vi "DI IRQ Preview.vi"(6 "Edge Count:":u32, 7 "Type:":T1, 8 "error in (no error)":errorcluster, 9 "_Count Label Refnum":refnum<vi>, 10 "_Counts Refnum":refnum<vi>, 11 "_Digtal Preview Refnum":refnum<vi>) -> (0 "error out":errorcluster)   [LabVIEW 2021]
uses:
  <vilib>/myRIO/Common/Instrument Driver Framework/myRIO v1.0/IRQ/typedefs/DI IRQ Type.ctl
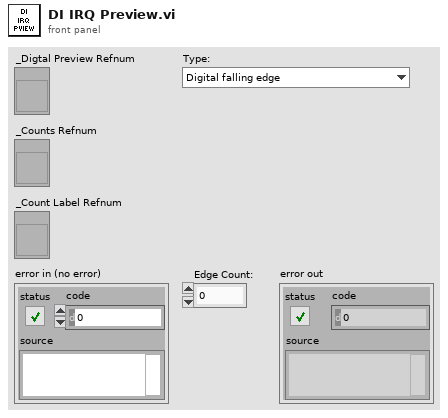
[diagram p1: front panel]
types:
  T1 = typedef "DI IRQ Type.ctl" = enum16{"Digital falling edge", "Digital rising edge", "Digital edge"}
  T2 = cluster{"Analog Preview 3":cluster{"X":dbl, "Y":dbl}[]}[]
  T3 = cluster{"Analog Preview 3":cluster{"X":dbl, "Y":dbl}[]}
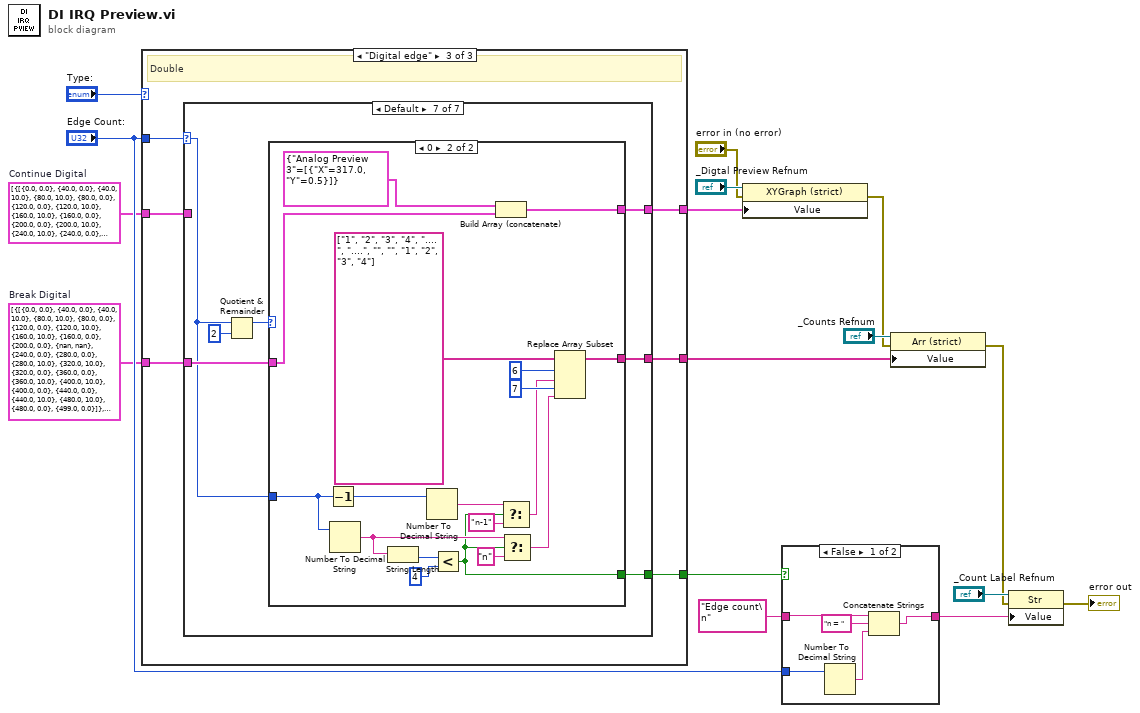
[diagram p0: block diagram]
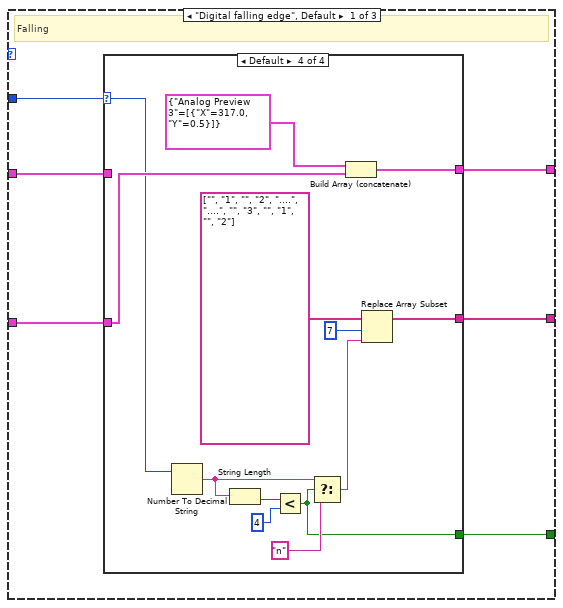
[diagram p3: hidden frame]
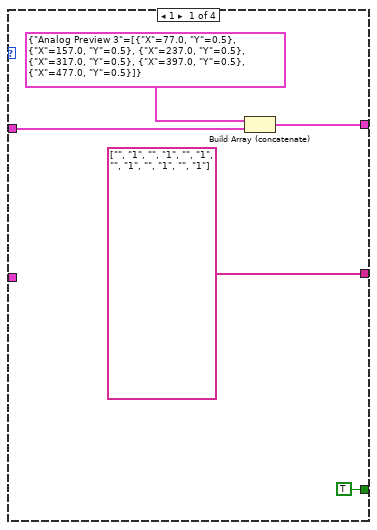
[diagram p4: hidden frame]
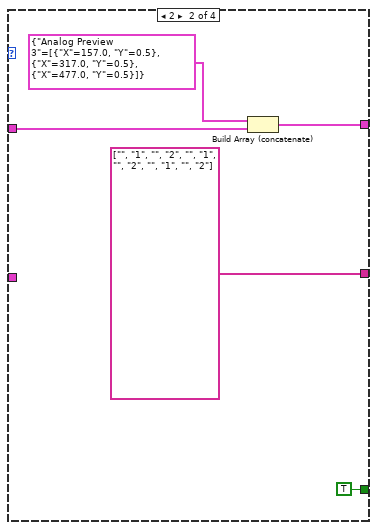
[diagram p5: hidden frame]
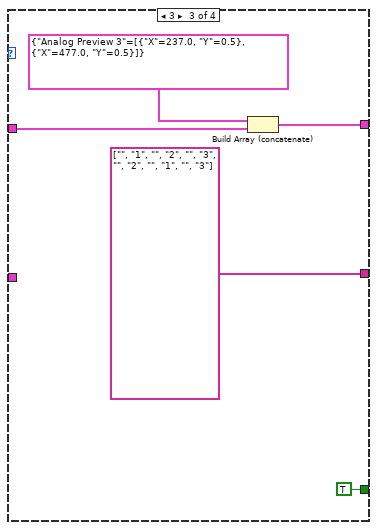
[diagram p6: hidden frame]
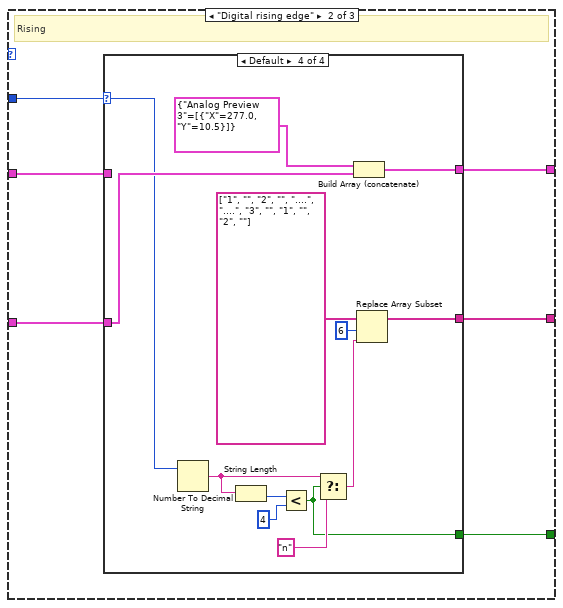
[diagram p7: hidden frame]
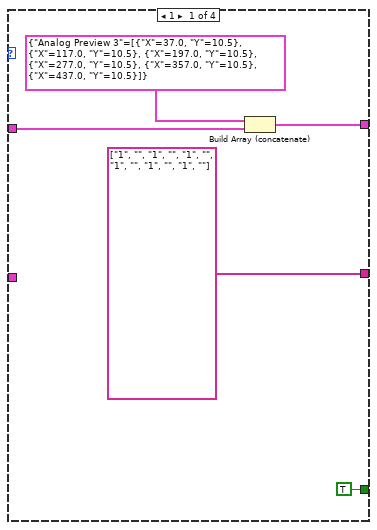
[diagram p8: hidden frame]
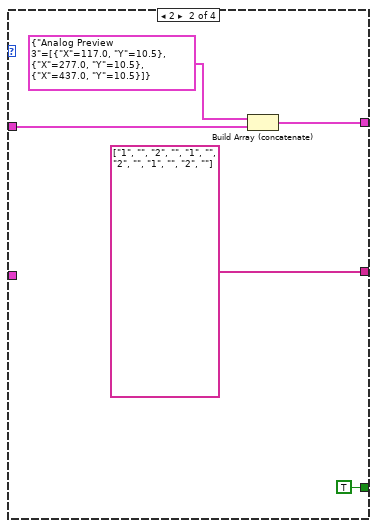
[diagram p9: hidden frame]
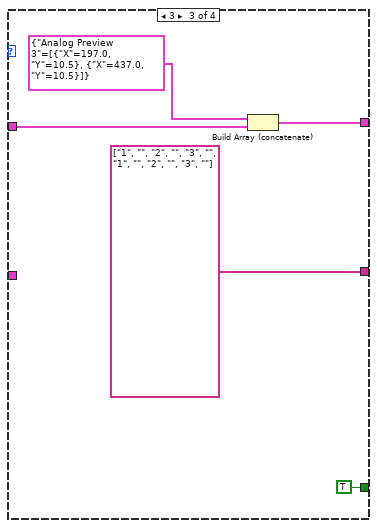
[diagram p10: hidden frame]
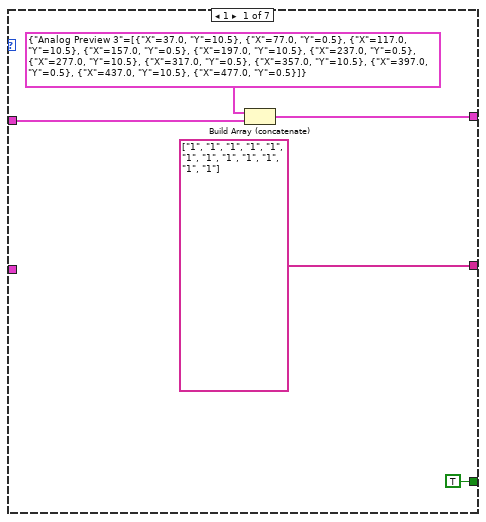
[diagram p11: hidden frame]
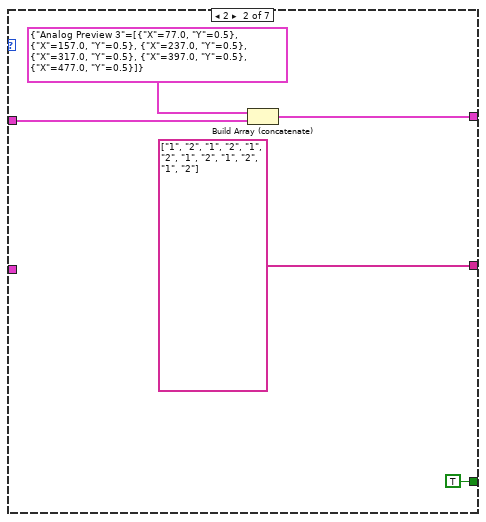
[diagram p12: hidden frame]
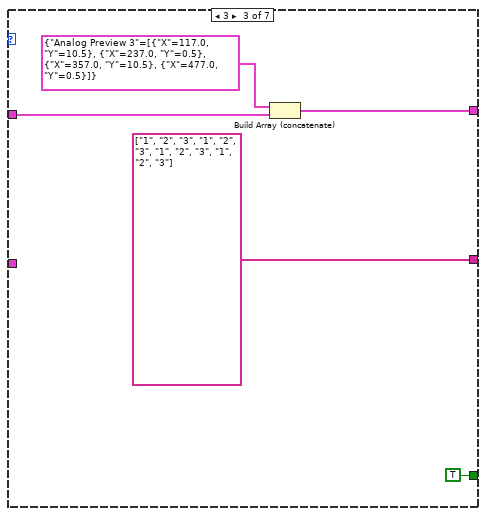
[diagram p13: hidden frame]
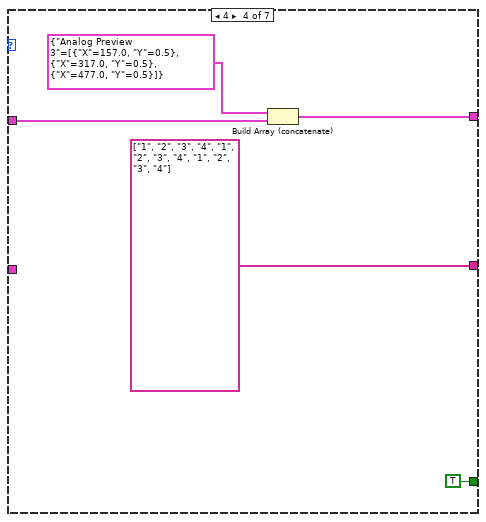
[diagram p14: hidden frame]
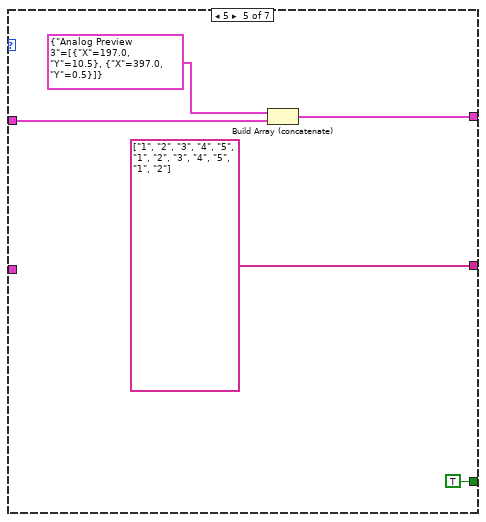
[diagram p15: hidden frame]
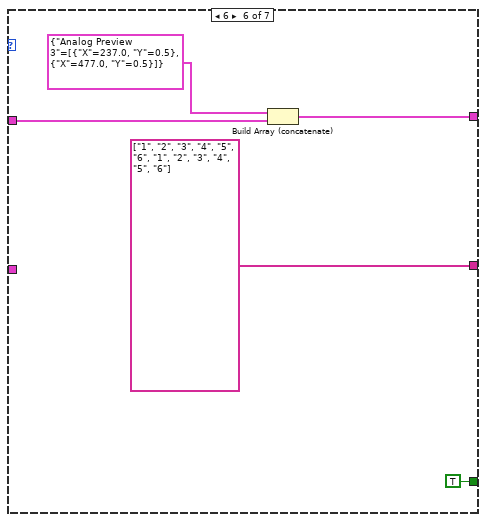
[diagram p16: hidden frame]
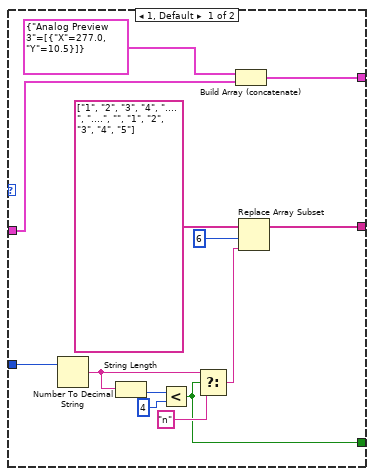
[diagram p17: hidden frame]
diagram:
  w8 = T2 [{"Analog Preview 3"=[{"X"=0.0, "Y"=0.0}, {"X"=40.0, "Y"=0.0}, {"X"=40.0, "Y"=10.0}, {"X"=80.0, "Y"=10.0}, {"X"=80.0, "Y"=0.0}, {"X"=120.0, "Y"=0.0}, {"X"=120.0, "Y"=10.0}, {"X"=160.0, "Y"=10.0}, {"X"=160.0, "Y"=0.0}, {"X"=200.0, "Y"=0.0}, {"X"=nan, "Y"=nan}, {"X"=240.0, "Y"=0.0}, {"X"=280.0, "Y"=0.0}, {"X"=280.0, "Y"=10.0}, {"X"=320.0, "Y"=10.0}, {"X"=320.0, "Y"=0.0}, {"X"=360.0, "Y"=0.0}, {"X"=360.0, "Y"=10.0}, {"X"=400.0, "Y"=10.0}, {"X"=400.0, "Y"=0.0}, {"X"=440.0, "Y"=0.0}, {"X"=440.0, "Y"=10.0}, {"X"=480.0, "Y"=10.0}, {"X"=480.0, "Y"=0.0}, {"X"=499.0, "Y"=0.0}]}, {"Analog Preview 3"=[{"X"=190.0, "Y"=-2.0}, {"X"=200.0, "Y"=0.0}, {"X"=190.0, "Y"=2.0}, {"X"=200.0, "Y"=4.0}, {"X"=nan, "Y"=nan}, {"X"=200.0, "Y"=-2.0}, {"X"=210.0, "Y"=0.0}, {"X"=200.0, "Y"=2.0}, {"X"=210.0, "Y"=4.0}, {"X"=nan, "Y"=nan}, {"X"=220.0, "Y"=-2.0}, {"X"=230.0, "Y"=0.0}, {"X"=220.0, "Y"=2.0}, {"X"=230.0, "Y"=4.0}, {"X"=nan, "Y"=nan}, {"X"=230.0, "Y"=-2.0}, {"X"=240.0, "Y"=0.0}, {"X"=230.0, "Y"=2.0}, {"X"=240.0, "Y"=4.0}]}]  # Break Digital
  w9 = T2 [{"Analog Preview 3"=[{"X"=0.0, "Y"=0.0}, {"X"=40.0, "Y"=0.0}, {"X"=40.0, "Y"=10.0}, {"X"=80.0, "Y"=10.0}, {"X"=80.0, "Y"=0.0}, {"X"=120.0, "Y"=0.0}, {"X"=120.0, "Y"=10.0}, {"X"=160.0, "Y"=10.0}, {"X"=160.0, "Y"=0.0}, {"X"=200.0, "Y"=0.0}, {"X"=200.0, "Y"=10.0}, {"X"=240.0, "Y"=10.0}, {"X"=240.0, "Y"=0.0}, {"X"=280.0, "Y"=0.0}, {"X"=280.0, "Y"=10.0}, {"X"=320.0, "Y"=10.0}, {"X"=320.0, "Y"=0.0}, {"X"=360.0, "Y"=0.0}, {"X"=360.0, "Y"=10.0}, {"X"=400.0, "Y"=10.0}, {"X"=400.0, "Y"=0.0}, {"X"=440.0, "Y"=0.0}, {"X"=440.0, "Y"=10.0}, {"X"=480.0, "Y"=10.0}, {"X"=480.0, "Y"=0.0}, {"X"=499.0, "Y"=0.0}]}]  # Continue Digital
  n1 = case shown="\"Digital edge\"" "Type:" {
    tunnel: "Edge Count:" -> [w22 w56 w86]
    tunnel: w9 -> [w21 w55 w90]
    tunnel: [w19 w54 w88] -> w14
    tunnel: [w18 w53 w87] -> w15
    tunnel: w8 -> [w20 w52 w89]
    tunnel: [w17 w51 w85] -> w11
    frame "Digital falling edge", Default {
      # "Falling"
      n2 = case shown="Default" w22 {
        selector: w22 -> [_ _ _ w40]
        tunnel: w21 -> [w27 w32 w36 _]
        tunnel: [w25 w31 w35 w48] -> w19
        tunnel: [string[] ["", "1", "", "1", "", "1", "", "1", "", "1", "", "1"] ("Count") string[] ["", "1", "", "2", "", "1", "", "2", "", "1", "", "2"] ("Count") string[] ["", "1", "", "2", "", "3", "", "2", "", "1", "", "3"] ("Count") w46] -> w18
        tunnel: w20 -> [_ _ _ w49]
        tunnel: [TRUE TRUE TRUE w38] -> w17
        frame 1 {
          n3 = Build Array (concatenate)(T3 {"Analog Preview 3"=[{"X"=77.0, "Y"=0.5}, {"X"=157.0, "Y"=0.5}, {"X"=237.0, "Y"=0.5}, {"X"=317.0, "Y"=0.5}, {"X"=397.0, "Y"=0.5}, {"X"=477.0, "Y"=0.5}]}, w27) -> (w25:T2)
        }
        frame 2 {
          n4 = Build Array (concatenate)(T3 {"Analog Preview 3"=[{"X"=157.0, "Y"=0.5}, {"X"=317.0, "Y"=0.5}, {"X"=477.0, "Y"=0.5}]}, w32) -> (w31:T2)
        }
        frame 3 {
          n5 = Build Array (concatenate)(T3 {"Analog Preview 3"=[{"X"=237.0, "Y"=0.5}, {"X"=477.0, "Y"=0.5}]}, w36) -> (w35:T2)
        }
        frame Default {
          n6 = Number To Decimal String(number=w40) -> (decimal integer string=w42:string)  [unwired: 1 in]
          n7 = String Length(string=w42) -> (length=w44:i32)
          n8 = Less?(x=w44, y=4) -> (x < y?=w38:bool)
          n9 = Select(t=w42, s=w38, f="n") -> (s? t:f=w39:string)
          n10 = Build Array (concatenate)(T3 {"Analog Preview 3"=[{"X"=317.0, "Y"=0.5}]}, w49) -> (w48:T2)
          n11 = Replace Array Subset(array=string[] ["", "1", "", "2", "....", "....", "", "3", "", "1", "", "2"] ("Count"), new element=w39, index=7) -> (w46:string[])
        }
      }
    }
    frame "Digital rising edge" {
      # "Rising"
      n12 = case shown="Default" w56 {
        selector: w56 -> [_ _ _ w78]
        tunnel: w55 -> [w61 w65 w70 _]
        tunnel: [w59 w64 w69 w82] -> w54
        tunnel: [string[] ["1", "", "1", "", "1", "", "1", "", "1", "", "1", ""] ("Count") string[] ["1", "", "2", "", "1", "", "2", "", "1", "", "2", ""] ("Count") string[] ["1", "", "2", "", "3", "", "1", "", "2", "", "3", ""] ("Count") w80] -> w53
        tunnel: w52 -> [_ _ _ w83]
        tunnel: [TRUE TRUE TRUE w72] -> w51
        frame 1 {
          n13 = Build Array (concatenate)(T3 {"Analog Preview 3"=[{"X"=37.0, "Y"=10.5}, {"X"=117.0, "Y"=10.5}, {"X"=197.0, "Y"=10.5}, {"X"=277.0, "Y"=10.5}, {"X"=357.0, "Y"=10.5}, {"X"=437.0, "Y"=10.5}]}, w61) -> (w59:T2)
        }
        frame 2 {
          n14 = Build Array (concatenate)(T3 {"Analog Preview 3"=[{"X"=117.0, "Y"=10.5}, {"X"=277.0, "Y"=10.5}, {"X"=437.0, "Y"=10.5}]}, w65) -> (w64:T2)
        }
        frame 3 {
          n15 = Build Array (concatenate)(T3 {"Analog Preview 3"=[{"X"=197.0, "Y"=10.5}, {"X"=437.0, "Y"=10.5}]}, w70) -> (w69:T2)
        }
        frame Default {
          n16 = Number To Decimal String(number=w78) -> (decimal integer string=w75:string)  [unwired: 1 in]
          n17 = String Length(string=w75) -> (length=w77:i32)
          n18 = Less?(x=w77, y=4) -> (x < y?=w72:bool)
          n19 = Select(t=w75, s=w72, f="n") -> (s? t:f=w74:string)
          n20 = Build Array (concatenate)(T3 {"Analog Preview 3"=[{"X"=277.0, "Y"=10.5}]}, w83) -> (w82:T2)
          n21 = Replace Array Subset(array=string[] ["1", "", "2", "", "....", "....", "3", "", "1", "", "2", ""] ("Count"), new element=w74, index=6) -> (w80:string[])
        }
      }
    }
    frame "Digital edge" {
      # "Double"
      n22 = case shown="Default" w86 {
        selector: w86 -> [_ _ _ _ _ _ w124]
        tunnel: w90 -> [w95 w100 w104 w109 w114 w119 _]
        tunnel: [w93 w99 w103 w108 w113 w118 w126] -> w88
        tunnel: [string[] ["1", "1", "1", "1", "1", "1", "1", "1", "1", "1", "1", "1"] ("Count") string[] ["1", "2", "1", "2", "1", "2", "1", "2", "1", "2", "1", "2"] ("Count") string[] ["1", "2", "3", "1", "2", "3", "1", "2", "3", "1", "2", "3"] ("Count") string[] ["1", "2", "3", "4", "1", "2", "3", "4", "1", "2", "3", "4"] ("Count") string[] ["1", "2", "3", "4", "5", "1", "2", "3", "4", "5", "1", "2"] ("Count") string[] ["1", "2", "3", "4", "5", "6", "1", "2", "3", "4", "5", "6"] ("Count") w125] -> w87
        tunnel: w89 -> [_ _ _ _ _ _ w127]
        tunnel: [TRUE TRUE TRUE TRUE TRUE TRUE w121] -> w85
        frame 1 {
          n23 = Build Array (concatenate)(T3 {"Analog Preview 3"=[{"X"=37.0, "Y"=10.5}, {"X"=77.0, "Y"=0.5}, {"X"=117.0, "Y"=10.5}, {"X"=157.0, "Y"=0.5}, {"X"=197.0, "Y"=10.5}, {"X"=237.0, "Y"=0.5}, {"X"=277.0, "Y"=10.5}, {"X"=317.0, "Y"=0.5}, {"X"=357.0, "Y"=10.5}, {"X"=397.0, "Y"=0.5}, {"X"=437.0, "Y"=10.5}, {"X"=477.0, "Y"=0.5}]}, w95) -> (w93:T2)
        }
        frame 2 {
          n24 = Build Array (concatenate)(T3 {"Analog Preview 3"=[{"X"=77.0, "Y"=0.5}, {"X"=157.0, "Y"=0.5}, {"X"=237.0, "Y"=0.5}, {"X"=317.0, "Y"=0.5}, {"X"=397.0, "Y"=0.5}, {"X"=477.0, "Y"=0.5}]}, w100) -> (w99:T2)
        }
        frame 3 {
          n25 = Build Array (concatenate)(T3 {"Analog Preview 3"=[{"X"=117.0, "Y"=10.5}, {"X"=237.0, "Y"=0.5}, {"X"=357.0, "Y"=10.5}, {"X"=477.0, "Y"=0.5}]}, w104) -> (w103:T2)
        }
        frame 4 {
          n26 = Build Array (concatenate)(T3 {"Analog Preview 3"=[{"X"=157.0, "Y"=0.5}, {"X"=317.0, "Y"=0.5}, {"X"=477.0, "Y"=0.5}]}, w109) -> (w108:T2)
        }
        frame 5 {
          n27 = Build Array (concatenate)(T3 {"Analog Preview 3"=[{"X"=197.0, "Y"=10.5}, {"X"=397.0, "Y"=0.5}]}, w114) -> (w113:T2)
        }
        frame 6 {
          n28 = Build Array (concatenate)(T3 {"Analog Preview 3"=[{"X"=237.0, "Y"=0.5}, {"X"=477.0, "Y"=0.5}]}, w119) -> (w118:T2)
        }
        frame Default {
          n29 = Quotient & Remainder(x=w124, y=u32 2) -> (x-y*floor(x/y)=w122:u32)  [unwired: 1 out]
          n30 = case shown="0" w122 {
            tunnel: w127 -> [w139 w157]
            tunnel: [w138 w156] -> w126
            tunnel: [w136 w154] -> w125
            tunnel: w124 -> [w130 w145]
            tunnel: [w128 w141] -> w121
            frame 1, Default {
              n31 = Number To Decimal String(number=w130) -> (decimal integer string=w132:string)  [unwired: 1 in]
              n32 = String Length(string=w132) -> (length=w134:i32)
              n33 = Less?(x=w134, y=4) -> (x < y?=w128:bool)
              n34 = Select(t=w132, s=w128, f="n") -> (s? t:f=w129:string)
              n35 = Build Array (concatenate)(T3 {"Analog Preview 3"=[{"X"=277.0, "Y"=10.5}]}, w139) -> (w138:T2)
              n36 = Replace Array Subset(array=string[] ["1", "2", "3", "4", "....", "....", "", "1", "2", "3", "4", "5"] ("Count"), new element=w129, index=6) -> (w136:string[])
            }
            frame 0 {
              n37 = Decrement(x=w145) -> (x-1=w151:u32)
              n38 = Number To Decimal String(number=w145) -> (decimal integer string=w148:string)  [unwired: 1 in]
              n39 = String Length(string=w148) -> (length=w150:i32)
              n40 = Number To Decimal String(number=w151) -> (decimal integer string=w144:string)  [unwired: 1 in]
              n41 = Less?(x=w150, y=4) -> (x < y?=w141:bool)
              n42 = Build Array (concatenate)(T3 {"Analog Preview 3"=[{"X"=317.0, "Y"=0.5}]}, w157) -> (w156:T2)
              n43 = Select(t=w144, s=w141, f="n-1") -> (s? t:f=w143:string)
              n44 = Select(t=w148, s=w141, f="n") -> (s? t:f=w146:string)
              n45 = Replace Array Subset(array=string[] ["1", "2", "3", "4", "....", "....", "", "", "1", "2", "3", "4"] ("Count"), new element #1=w143, index #1=6 ("index"), new element #2=w146, index #2=7 ("index")) -> (w154:string[])
            }
          }
        }
      }
    }
  }
  n46 = property on="Property Node" class="XYGraph (strict)"(reference="_Digtal Preview Refnum", error in="error in (no error)", "Value"=w14) -> (error out=w2:errorcluster)  [unwired: 1 out]
  n47 = case shown="False" w11 {
    tunnel: [w159 w164] -> w16
    tunnel: "Edge count\n" ("Hysteresis") -> [w163 w164]
    tunnel: "Edge Count:" -> [w160 _]
    frame False {
      n48 = Number To Decimal String(number=w160) -> (decimal integer string=w161:string)  [unwired: 1 in]
      n49 = Concatenate Strings(w163, "n = " ("string"), w161) -> (w159:string)
    }
    frame True {
    }
  }
  n50 = property on="Property Node" class="Arr (strict)"(reference="_Counts Refnum", error in=w2, "Value"=w15) -> (error out=w1:errorcluster)  [unwired: 1 out]
  n51 = property on="Property Node" class="Str"(reference="_Count Label Refnum", error in=w1, "Value"=w16) -> (error out=→"error out":errorcluster)  [unwired: 1 out]
